vi "Create Database.vi"(8 "error in (no error)":errorcluster, 10 "Database Configuration":T1={"Interface"="CAN1", "CAN Cluster"={"Baud Rate"=125000, "Comment"="", "Name"="CAN_Cluster"}, "CAN Frame"={"Frame name"="frame1", "Identifier"=1, "Payload Length"=8, "Timing Type"=1, "Transmit Time"=0.0, "Extended Identifier?"=FALSE, "Comment"=""}, "Signal Cluster"={"Signal name"="signal", "Scaling Factor"=1.0, "Scaling Offset"=0.0, "Maximum Value"=256.0, "Minimum Value"=0.0, "Default Value"=0.0, "Unit"="V", "Start Bit"=0, "Number of Bits"=8, "Data Type"=1, "Byte Order"=0, "Comment"=""}, "Session Type (All Single Point)"=enum."Signal Input"} {"Signal Cluster"."Byte Order" items=["Little Endian", "Big Endian"]; "Signal Cluster"."Data Type" items=["Signed", "Unsigned", "IEEE Float"]; "CAN Frame"."Timing Type" items=["Cyclic Data", "Event Data", "Cyclic Remote", "Event Remote"]}, 11 "Abstract in":refnum<class "Abstract.lvclass">) -> (0 "error out":errorcluster, 3 "Abstract out":refnum<class "Abstract.lvclass">)   [LabVIEW 2021, in "CAN.lvlib" / "Abstract.lvclass"]
uses:
  Abstract.lvclass
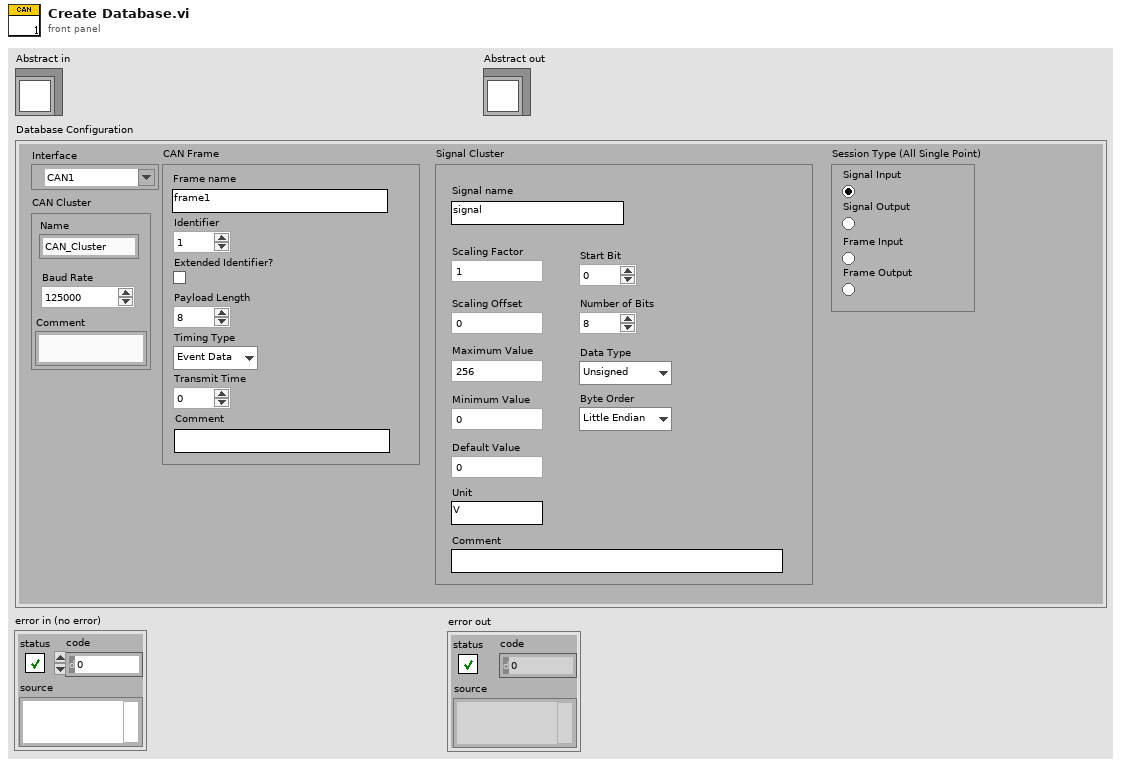
[diagram p1: front panel]
types:
  T1 = cluster{"Interface":refnum<k21>, "CAN Cluster":cluster{"Baud Rate":u32, "Comment":string, "Name":string}, "CAN Frame":cluster{"Frame name":string, "Identifier":u32, "Payload Length":u32, "Timing Type":u32, "Transmit Time":dbl, "Extended Identifier?":bool, "Comment":string}, "Signal Cluster":cluster{"Signal name":string, "Scaling Factor":dbl, "Scaling Offset":dbl, "Maximum Value":dbl, "Minimum Value":dbl, "Default Value":dbl, "Unit":string, "Start Bit":u32, "Number of Bits":u32, "Data Type":u32, "Byte Order":u32, "Comment":string}, "Session Type (All Single Point)":enum32{"Signal Input", "Signal Output", "Frame Input", "Frame Output"}}
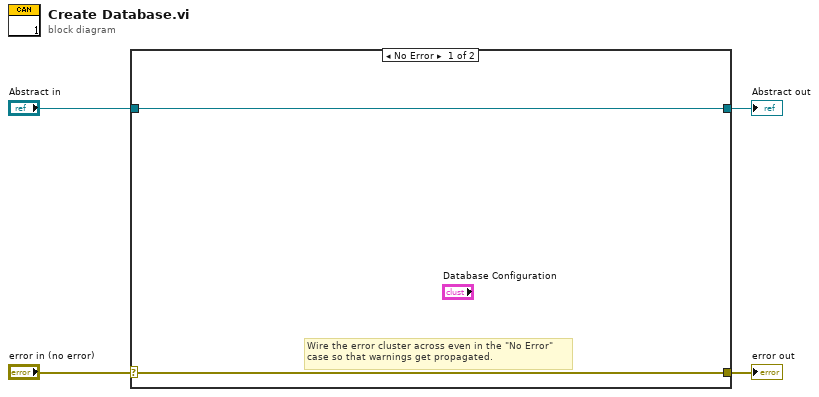
[diagram p0: block diagram]
diagram:
  n1 = case shown="No Error" "error in (no error)" {
    selector: "error in (no error)" -> [w5 w8]
    tunnel: [w5 w8] -> w3
    tunnel: [w6 w7] -> w1
    tunnel: "Abstract in" -> [w6 w7]
    frame No Error {
      # "Wire the error cluster across even in the \"No Error\"\ncase so that warnings get propagated."
    }
    frame Error {
    }
  }
  "error out" <- w3
  "Abstract out" <- w1
